vi "LEP_RV_SanityCheck.vi"(8 "error in (no error)":errorcluster, 11 "display dialog? (T)":bool=TRUE) -> (0 "error out":errorcluster, 3 "ok":bool)   [LabVIEW 2011]
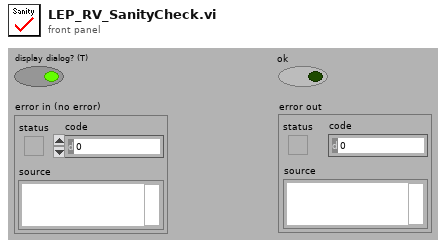
[diagram p1: front panel]
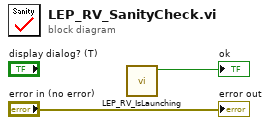
[diagram p0: block diagram]
diagram:
  n1 = call "LEP_RV_IsLaunching.vi"() -> ("not in memory"=→"ok":bool)  [unwired: 11 in]
  "error out" <- "error in (no error)"
